vi "BPSK_Convcode.vi"(5 "EN_Convcode":dbl, 8 "error in":errorcluster, 10 "input_data":dbl[](array[numeric]), 11 "Path In":path) -> (0 "error out":errorcluster, 2 "output_data":dbl[](array[numeric]), 3 "Path Out":path)   [LabVIEW 2015]
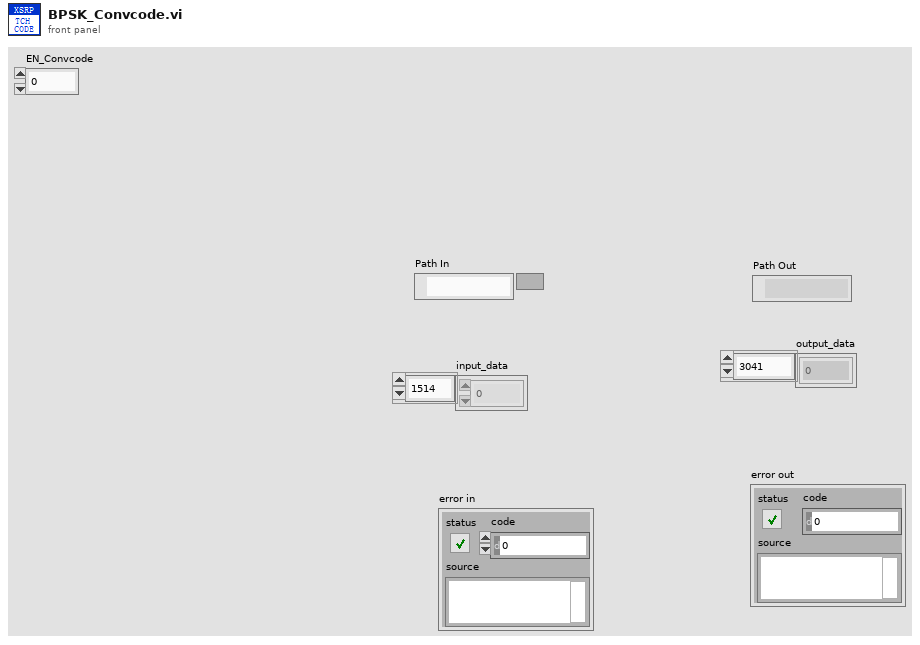
[diagram p1: front panel]
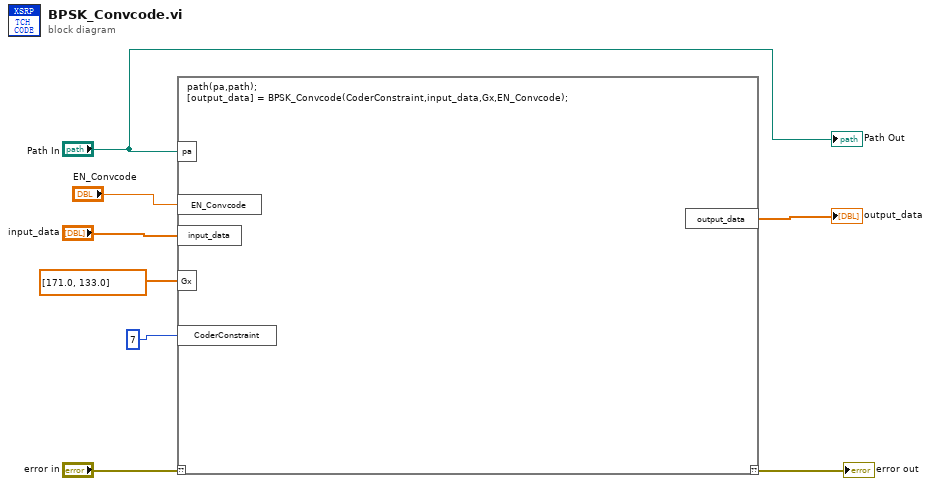
[diagram p0: block diagram]
diagram:
  n1 = script code="path(pa,path);\n[output_data] = BPSK_Convcode(CoderConstraint,input_data,Gx,EN_Convcode);"("??"="error in", "pa"="Path In", "input_data"="input_data", "Gx"=dbl[] [171.0, 133.0], "CoderConstraint"=7, "EN_Convcode"="EN_Convcode") -> ("??"=→"error out":errorcluster, "output_data"=→"output_data":dbl[])
  "Path Out" <- "Path In"
